vi "Discovery Client FGV.vi"(8 "error in":errorcluster, 10 "unique id in":u64, 11 "action":T2) -> (0 "error out":errorcluster, 2 "unique id out":u64, 3 "grpc client id":T1)   [LabVIEW 2020, in "MeasurementLink Discovery V1.lvlib"]
uses:
  MeasurementLink Discovery V1.lvlib
  TypeDefs/gRPC Client Cache FGV Action.ctl
  <vilib>/gRPC/LabVIEW gRPC Library/Shared/grpcId.ctl
  TypeDefs/gRPC Client Cache VI References.ctl
  <vilib>/gRPC/LabVIEW gRPC Library/grpc-lvsupport-release.lvlib
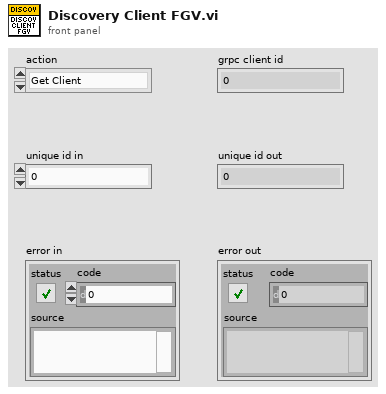
[diagram p1: front panel]
types:
  T1 = typedef "grpc-lvsupport-release.lvlib/grpcId.ctl" = u64
  T2 = typedef "MeasurementLink Discovery V1.lvlib/gRPC Client Cache FGV Action.ctl" = enum16{"Get Client", "Recreate Client"}
  T3 = typedef "MeasurementLink Discovery V1.lvlib/gRPC Client Cache VI References.ctl" = cluster{"create vi reference":refnum<vi>, "recreate vi reference":refnum<vi>}
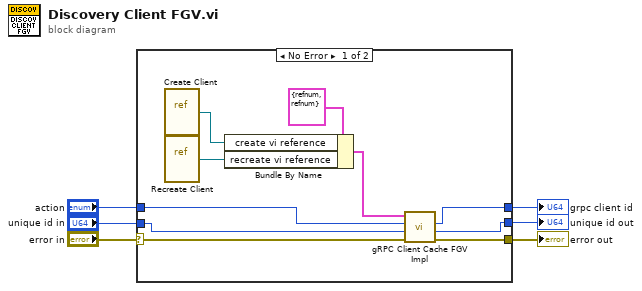
[diagram p0: block diagram]
diagram:
  n1 = case shown="No Error" "error in" {
    selector: "error in" -> [w16 w17]
    tunnel: [w13 w17] -> w6
    tunnel: "action" -> [w15 _]
    tunnel: [w12 _] -> w5
    tunnel: "unique id in" -> [w14 _]
    tunnel: [w11 _] -> w1
    frame No Error {
      n2 = vi-ref "Create Client.vi"() -> (w9:refnum<vi>)
      n3 = vi-ref "Recreate Client.vi"() -> (w7:refnum<vi>)
      n4 = Bundle By Name(cluster=T3 {"create vi reference"=refnum, "recreate vi reference"=refnum} ("vi references in"), "create vi reference"=w9, "recreate vi reference"=w7) -> (w8:T3)
      n5 = call "gRPC Client Cache FGV Impl.vi"("error in"=w16, "unique id in"=w14, "action"=w15, "vi references in"=w8) -> ("error out"=w13:errorcluster, "unique id out"=w11:u64, "grpc client id"=w12:T1)  [unwired: 5 in]
    }
    frame Error {
    }
  }
  "error out" <- w6
  "grpc client id" <- w5
  "unique id out" <- w1
